vi "Get All Contexts.vi"() -> ()   [LabVIEW 2017]
panel:
  out "Application:Context Name":string
  out "size(s)":i32
  out "All Context Names":string[](array[string])
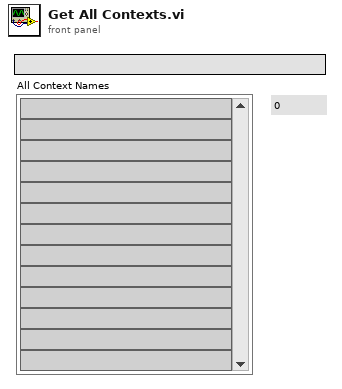
[diagram p1: front panel]
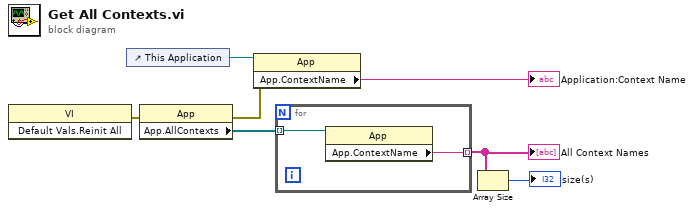
[diagram p0: block diagram]
diagram:
  n1 = invoke class="VI" method="Default Vals.Reinit All"() -> (error out=w2:errorcluster)  [unwired: 3 in, 2 out]
  n2 = control-ref of="This Application"() -> (w4:refnum<vi>)
  n3 = property class="App"(error in=w2) -> (error out=w1:errorcluster, "App.AllContexts"=w7:refnum<vi>[])  [unwired: 1 in, 1 out]
  n4 = property class="App"(reference=w4, error in=w1) -> ("App.ContextName"=→"Application:Context Name":string)  [unwired: 2 out]
  n5 = for {
    tunnel: w7 -> [w9] mode=indexing
    tunnel: [w8] -> w6 mode=indexing
    n6 = property class="App"(reference=w9) -> ("App.ContextName"=w8:string)  [unwired: 1 in, 2 out]
  }
  "All Context Names" <- w6
  n7 = Array Size(array=w6) -> (size(s)=→"size(s)":i32)
